vi "APC_PID_VariableMapping.vi"(3 "Index of array for 9056":i32[](array[numeric]), 4 "Index of array for 9049":i32[](array[numeric]), 5 "9056 IO":dbl[](array[numeric]), 6 "9049_CycleAveragedVariables":dbl[](array[numeric])) -> (0 "Index 9056":i32[](array[numeric]), 1 "Index 9049":i32[](array[numeric]), 2 "Output cluster":T1 caption="Visualization cluster")   [LabVIEW 2020]
uses:
  controls/APC_PIDCluster.ctl
  <vilib>/regexp/Match Regular Expression.xnode
  <vilib>/Utility/Data Type/NI_Data Type.lvlib
panel:
  out "Error Out 3":errorcluster
  in  "Ignore case":bool
  out "Element":string
  out "Error Out":errorcluster
  in  "Error In":errorcluster
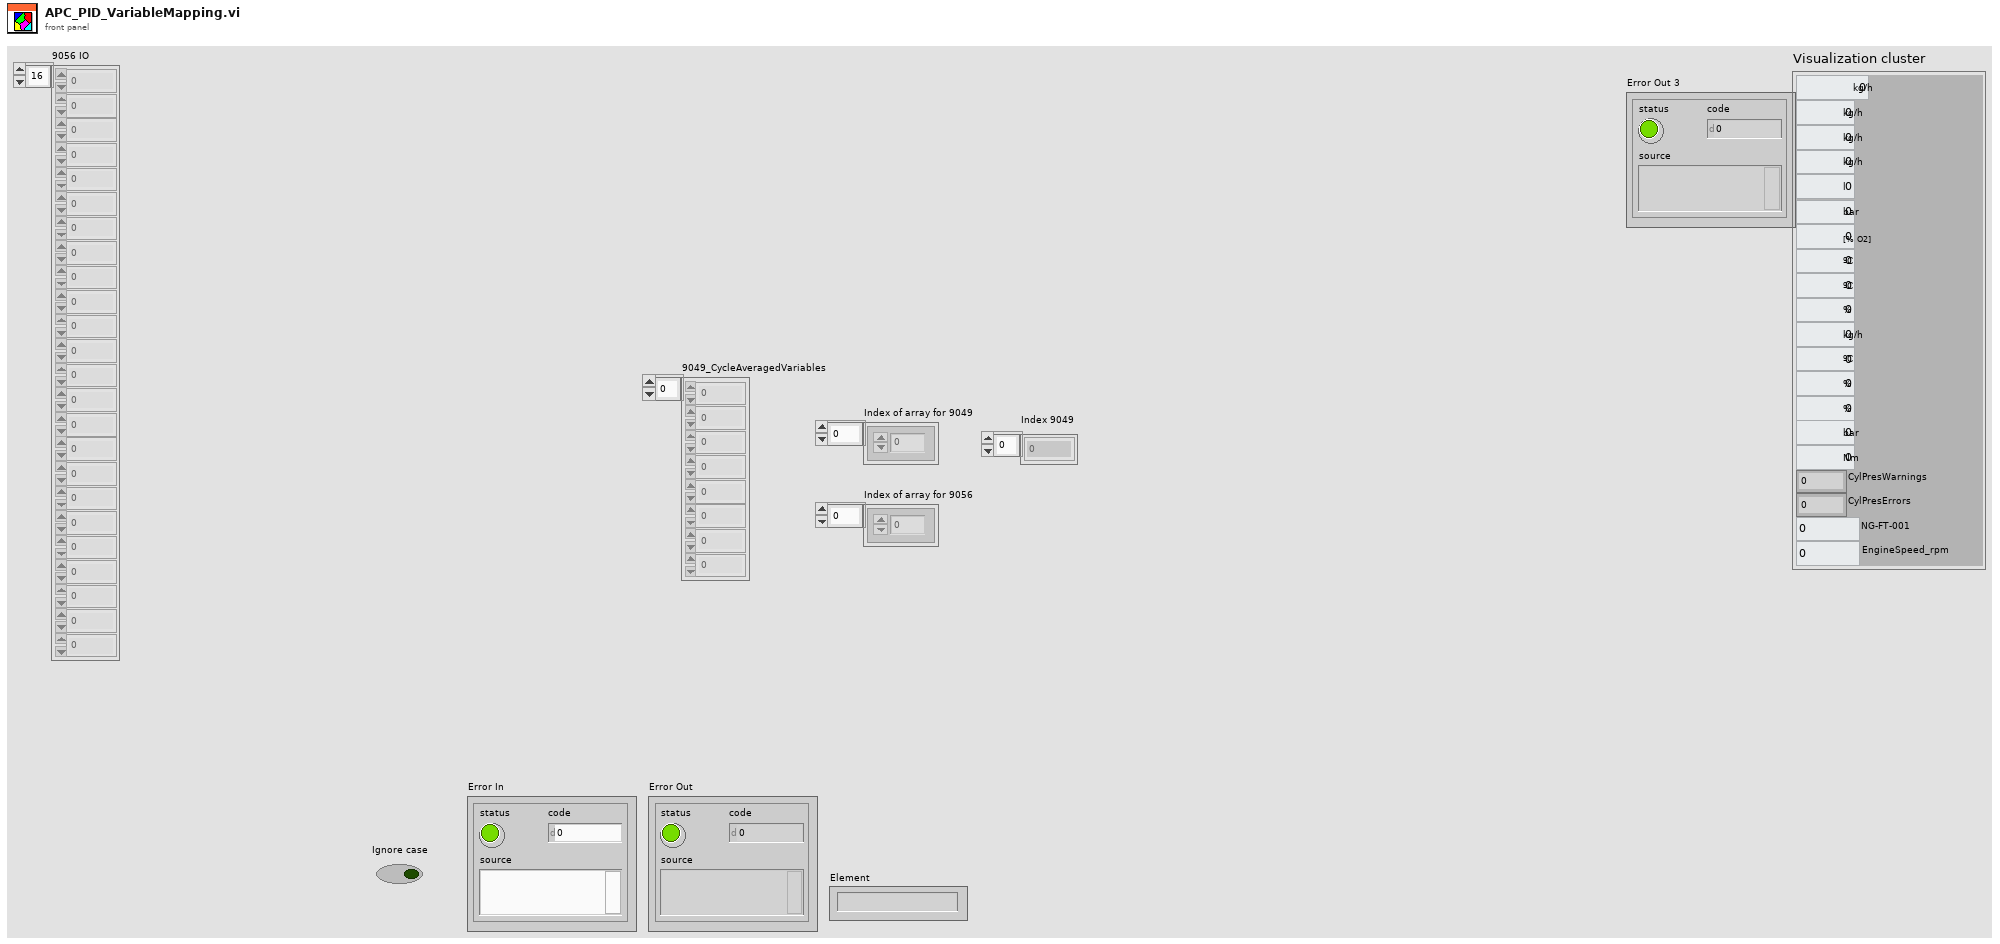
[diagram p1: front panel]
types:
  T1 = typedef "APC_PIDCluster.ctl" = cluster{"AR-FT-001":dbl, "O2-FC-001":dbl, "SW-FT-004":dbl, "SW-FT-002":dbl, "WF-OA-002":dbl, "WF-PT-004":dbl, "WF-OA-001":dbl, "EC-TT-001":dbl, "WF-TT-004":dbl, "EC-FC-001":dbl, "NG-FC-001":dbl, "EO-TT-001":dbl, "SW-FC-008":dbl, "SW-FC-004":dbl, "IMEPn6":dbl, "TORQUE":dbl, "CylPresWarnings":dbl, "CylPresErrors":dbl, "NG-FT-001":dbl, "EngineSpeed_rpm":dbl}
  T2 = cluster{"[0]":dbl, "[1]":dbl, "[2]":dbl, "[3]":dbl, "[4]":dbl, "[5]":dbl, "[6]":dbl, "[7]":dbl, "[8]":dbl, "[9]":dbl, "[10]":dbl, "[11]":dbl, "[12]":dbl, "[13]":dbl, "[14]":dbl, "[15]":dbl, "[16]":dbl, "[17]":dbl, "[18]":dbl, "[19]":dbl, "[20]":dbl, "[21]":dbl, "[22]":dbl, "[23]":dbl, "[24]":dbl, "[25]":dbl, "[26]":dbl, "[27]":dbl, "[28]":dbl, "[29]":dbl, "[30]":dbl, "[31]":dbl, "[32]":dbl, "[33]":dbl, "[34]":dbl, "[35]":dbl, "[36]":dbl, "[37]":dbl, "[38]":dbl, "[39]":dbl, "[40]":dbl, "[41]":dbl, "[42]":dbl, "[43]":dbl, "[44]":dbl, "[45]":dbl, "[46]":dbl, "[47]":dbl, "[48]":dbl, "[49]":dbl, "[50]":dbl, "[51]":dbl, "[52]":dbl, "[53]":dbl, "[54]":dbl, "[55]":dbl, "[56]":dbl, "[57]":dbl, "[58]":dbl, "[59]":dbl, "[60]":dbl, "[61]":dbl, "[62]":dbl, "[63]":dbl, "[64]":dbl, "[65]":dbl, "[66]":dbl, "[67]":dbl, "[68]":dbl, "[69]":dbl, "[70]":dbl, "[71]":dbl, "[72]":dbl, "[73]":dbl, "[74]":dbl, "[75]":dbl, "[76]":dbl, "[77]":dbl, "[78]":dbl, "[79]":dbl, "[80]":dbl, "[81]":dbl, "[82]":dbl, "[83]":dbl, "[84]":dbl, "[85]":dbl, "[86]":dbl, "[87]":dbl, "[88]":dbl, "[89]":dbl, "[90]":dbl, "[91]":dbl, "[92]":dbl, "[93]":dbl, "[94]":dbl, "[95]":dbl, "[96]":dbl, "[97]":dbl, "[98]":dbl, "[99]":dbl}
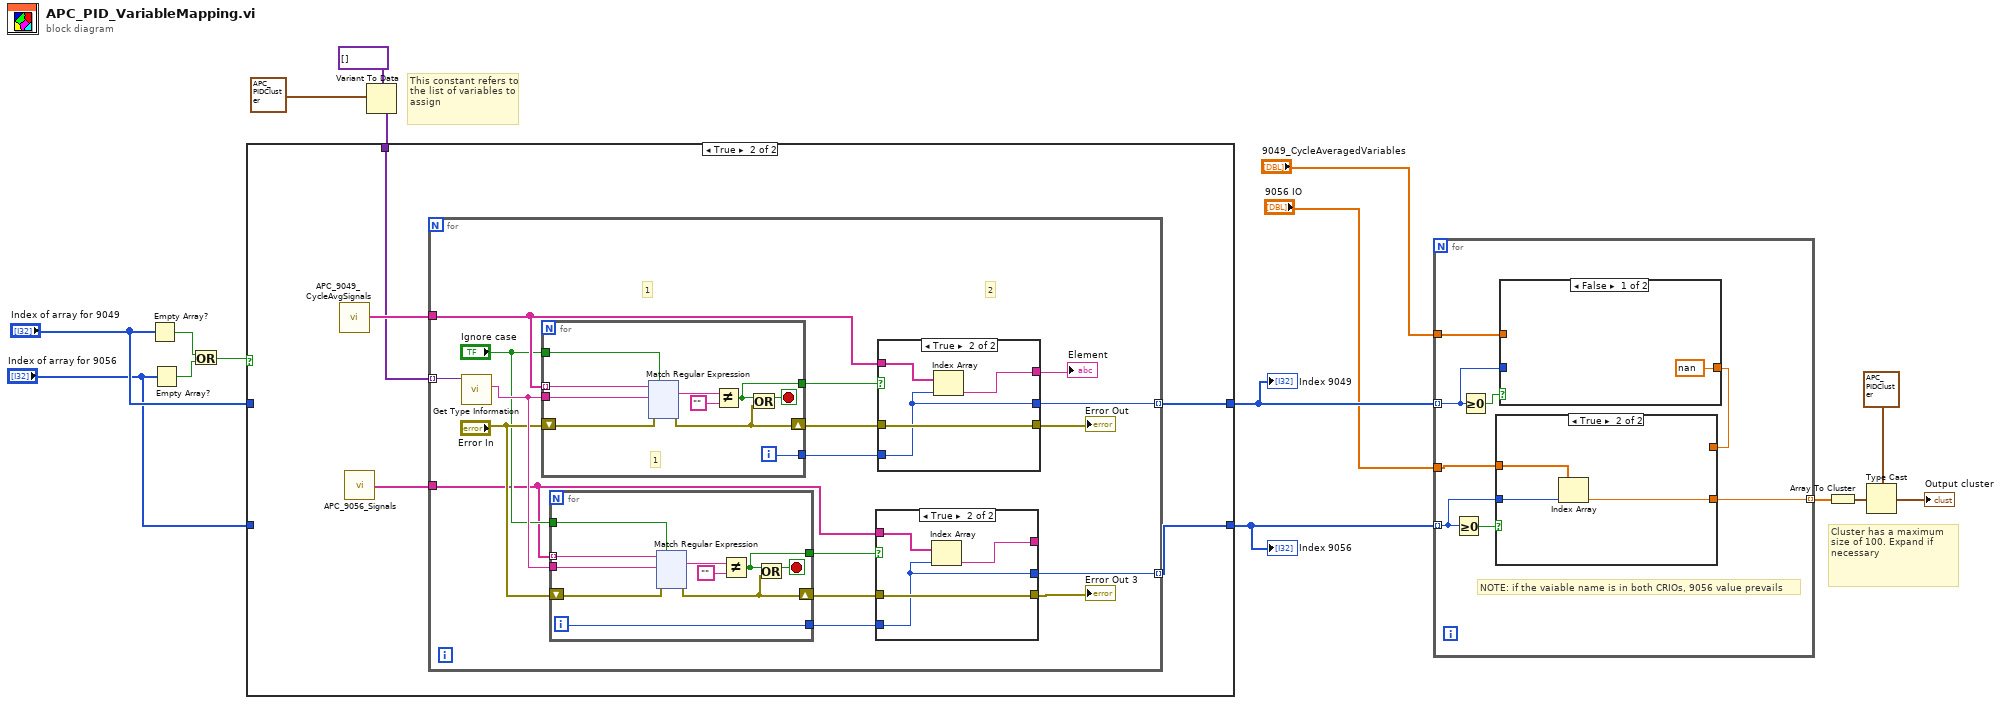
[diagram p0: block diagram]
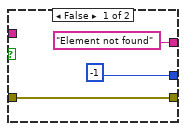
[diagram p3: hidden frame]
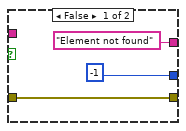
[diagram p4: hidden frame]
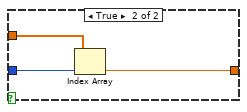
[diagram p6: hidden frame]
diagram:
  # "Cluster has a maximum size of 100. Expand if necessary"
  # "This constant refers to the list of variables to assign"
  n1 = Empty Array?(array="Index of array for 9049") -> (empty?=w10:bool)
  n2 = Empty Array?(array="Index of array for 9056") -> (empty?=w11:bool)
  n3 = Or(x=w10, y=w11) -> (x .or. y?=w9:bool)
  n4 = Variant To Data(type=variant[] [], Variant=T1 {"AR-FT-001"=0.0, "O2-FC-001"=0.0, "SW-FT-004"=0.0, "SW-FT-002"=0.0, "WF-OA-002"=0.0, "WF-PT-004"=0.0, "WF-OA-001"=0.0, "EC-TT-001"=0.0, "WF-TT-004"=0.0, "EC-FC-001"=0.0, "NG-FC-001"=0.0, "EO-TT-001"=0.0, "SW-FC-008"=0.0, "SW-FC-004"=0.0, "IMEPn6"=0.0, "TORQUE"=0.0, "CylPresWarnings"=0.0, "CylPresErrors"=0.0, "NG-FT-001"=0.0, "EngineSpeed_rpm"=0.0} ("Visualization cluster")) -> (data=w12:variant[])  [unwired: 1 in, 1 out]
  n5 = case shown="True" w9 {
    tunnel: "Index of array for 9049" -> [w18 _]
    tunnel: [w18 w23] -> w15
    tunnel: w12 -> [_ w21]
    tunnel: "Index of array for 9056" -> [w17 _]
    tunnel: [w17 w19] -> w7
    frame False {
    }
    frame True {
      n6 = call "APC_9049_CycleAvgSignals.vi"() -> ("CRIo9049_CycleAvgSignals"=w22:string[])  [unwired: 3 in]
      n7 = call "APC_9056_Signals.vi"() -> ("9056_raster"=w20:string[])  [unwired: 3 in, 2 out]
      n8 = for {
        tunnel: w22 -> [w35]
        tunnel: [w34] -> w23 mode=indexing
        tunnel: w21 -> [w33] mode=indexing
        tunnel: w20 -> [w26]
        tunnel: [w24] -> w19 mode=indexing
        # "1"
        # "2"
        # "1"
        n9 = call <vilib>:"Get Type Information.vi"("variant"=w33) -> ("name"=w32:string)  [unwired: 6 in, 4 out]
        n10 = for {
          tunnel: w35 -> [w185] mode=indexing
          tunnel: [w182] -> w38
          tunnel: w32 -> [w183]
          shift-right: [w176] -> w37
          shift-left: "Error In" -> [w177]
          tunnel: [w180] -> w39
          tunnel: "Ignore case" -> [w178]
          i -> [w182]
          stop <- w179 stop-if-true
          n11 = xnode "Match Regular Expression"("input string"=w185, "regular expression"=w183, "error in"=w177, "ignore case? (F)"=w178) -> ("whole match"=w184:string, "error out"=w176:errorcluster)  [unwired: 2 in, 3 out]
          n12 = Not Equal?(x=w184, y="") -> (x != y?=w180:bool)
          n13 = Or(x=w180, y=w176) -> (x .or. y?=w179:bool)
        }
        n14 = for {
          tunnel: w26 -> [w57] mode=indexing
          tunnel: [w54] -> w25
          tunnel: w32 -> [w55]
          shift-right: [w48] -> w28
          shift-left: "Error In" -> [w49]
          tunnel: [w52] -> w29
          tunnel: "Ignore case" -> [w50]
          i -> [w54]
          stop <- w51 stop-if-true
          n15 = xnode "Match Regular Expression"("input string"=w57, "regular expression"=w55, "error in"=w49, "ignore case? (F)"=w50) -> ("whole match"=w56:string, "error out"=w48:errorcluster)  [unwired: 2 in, 3 out]
          n16 = Not Equal?(x=w56, y="") -> (x != y?=w52:bool)
          n17 = Or(x=w52, y=w48) -> (x .or. y?=w51:bool)
        }
        n18 = case shown="True" w29 {
          tunnel: w25 -> [_ w44]
          tunnel: w26 -> [_ w47]
          tunnel: ["Element not found" ("String") w46] -> _
          tunnel: [-1 w44] -> w24
          tunnel: w28 -> [w41 w45]
          tunnel: [w41 w45] -> w27
          frame False {
          }
          frame True {
            n19 = Index Array(array=w47, index=w44) -> (element=w46:string)
          }
        }
        "Error Out 3" <- w27
        n20 = case shown="True" w39 {
          tunnel: w38 -> [_ w172]
          tunnel: w35 -> [_ w175]
          tunnel: ["Element not found" ("String") w174] -> w40
          tunnel: [-1 w172] -> w34
          tunnel: w37 -> [w169 w173]
          tunnel: [w169 w173] -> w36
          frame False {
          }
          frame True {
            n21 = Index Array(array=w175, index=w172) -> (element=w174:string)
          }
        }
        "Error Out" <- w36
        "Element" <- w40
      }
    }
  }
  "Index 9049" <- w15
  "Index 9056" <- w7
  n22 = for {
    tunnel: w15 -> [w301] mode=indexing
    tunnel: "9049_CycleAveragedVariables" -> [w304]
    tunnel: w7 -> [w300] mode=indexing
    tunnel: "9056 IO" -> [w303]
    tunnel: [w297] -> w4 mode=indexing
    # "NOTE: if the vaiable name is in both CRIOs, 9056 value prevails"
    n23 = Greater Or Equal To 0?(x=w300) -> (x >= 0?=w299:bool)
    n24 = Greater Or Equal To 0?(x=w301) -> (x >= 0?=w302:bool)
    n25 = case shown="False" w302 {
      tunnel: w304 -> [_ w312]
      tunnel: w301 -> [_ w311]
      tunnel: [nan ("millisecond timer value") w310] -> w298
      frame False {
      }
      frame True {
        n26 = Index Array(array=w312, index=w311) -> (element=w310:dbl)
      }
    }
    n27 = case shown="True" w299 {
      tunnel: w303 -> [_ w308]
      tunnel: w300 -> [_ w307]
      tunnel: [w305 w306] -> w297
      tunnel: w298 -> [w305 _]
      frame False {
      }
      frame True {
        n28 = Index Array(array=w308, index=w307) -> (element=w306:dbl)
      }
    }
  }
  n29 = Array To Cluster(array=w4) -> (cluster=w5:T2)
  n30 = Type Cast(type=T1 {"AR-FT-001"=0.0, "O2-FC-001"=0.0, "SW-FT-004"=0.0, "SW-FT-002"=0.0, "WF-OA-002"=0.0, "WF-PT-004"=0.0, "WF-OA-001"=0.0, "EC-TT-001"=0.0, "WF-TT-004"=0.0, "EC-FC-001"=0.0, "NG-FC-001"=0.0, "EO-TT-001"=0.0, "SW-FC-008"=0.0, "SW-FC-004"=0.0, "IMEPn6"=0.0, "TORQUE"=0.0, "CylPresWarnings"=0.0, "CylPresErrors"=0.0, "NG-FT-001"=0.0, "EngineSpeed_rpm"=0.0} ("Visualization cluster"), x=w5) -> (*(type *) &x=→"Output cluster":T1)
